vi "Choreo_Trajectory_GetTotalTime.vi"(11 "ChoreoTrajectory":T1) -> (3 "TotalTime":dbl)   [LabVIEW 2019]
doc: "Return total time duration of this trajectory\n\nInputs: \n - ChoreoTrajectory - cluster - Input trajectory\n\nOutputs:\n - TotalTime - double - The total time duration of this trajectory.\n."
uses:
  TypeDef/ChoreoTrajectory.ctl
  TypeDef/ChoreoTrajectoryState.ctl
  ChoreoLib.lvlib
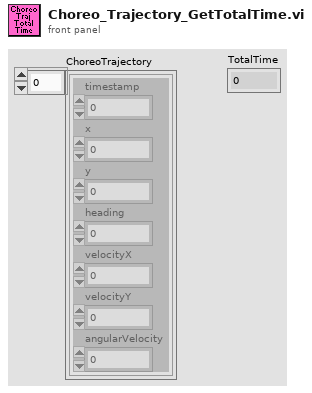
[diagram p1: front panel]
types:
  T1 = typedef "ChoreoLib.lvlib/ChoreoTrajectory.ctl" = T2[]
  T2 = typedef "ChoreoLib.lvlib/ChoreoTrajectoryState.ctl" = cluster{"timestamp":dbl, "x":dbl, "y":dbl, "heading":dbl, "velocityX":dbl, "velocityY":dbl, "angularVelocity":dbl}
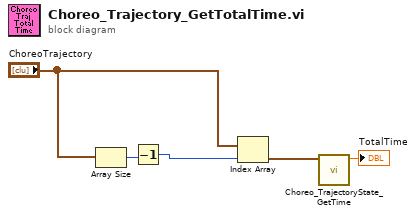
[diagram p0: block diagram]
diagram:
  n1 = Array Size(array="ChoreoTrajectory") -> (size(s)=w4:i32)
  n2 = Decrement(x=w4) -> (x-1=w3:i32)
  n3 = Index Array(array="ChoreoTrajectory", index=w3) -> (element=w2:T2)
  n4 = call "Choreo_TrajectoryState_GetTime.vi"("ChoreoTrajectoryState"=w2) -> ("timestamp"=→"TotalTime":dbl)  [unwired: 10 in]
